vi "Translate Data to Virtual Device Data.vi"(10 "HVAC Data":T1) -> (1 "Data Array":u16[](array[numeric]), 2 "Address":u16)   [LabVIEW 2015, in "SLZ-KA1 Actor.lvlib" / "SLZ-KA1.lvclass"]
doc: "This code converts the data coming from the real device to the format the EMS understands."
uses:
  SLZ-KA1.lvclass
  Controls/SLZ-KA1 Real Data Cluster.ctl
  Utilities/Modbus Data Conversion.llb/Modbus Data Conversion.lvlib
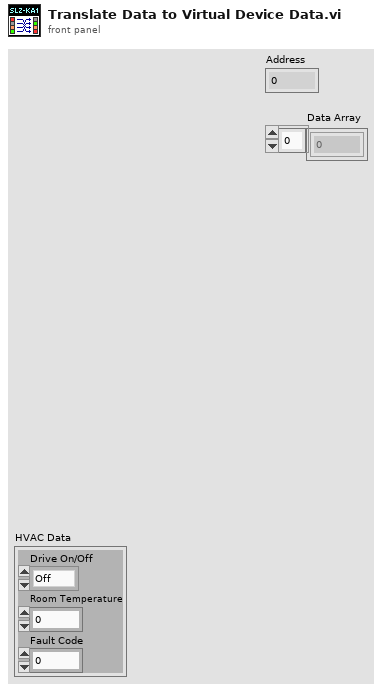
[diagram p1: front panel]
types:
  T1 = typedef "SLZ-KA1 Actor.lvlib/SLZ-KA1.lvclass/SLZ-KA1 Real Data Cluster.ctl" = cluster{"Drive On/Off":enum16{"Off", "On"}, "Room Temperature":dbl, "Fault Code":u16}
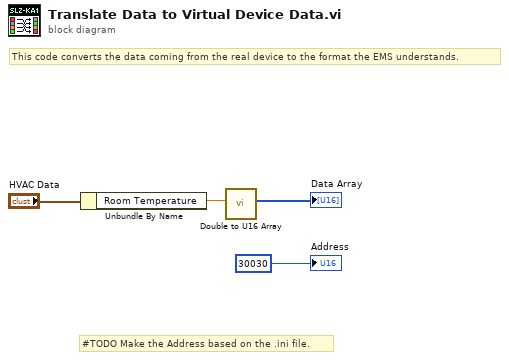
[diagram p0: block diagram]
diagram:
  # "This code converts the data coming from the real device to the format the EMS understands."
  # "#TODO Make the Address based on the .ini file."
  n1 = Unbundle By Name("HVAC Data") -> ("Room Temperature"=w1:dbl)
  n2 = call "Double to U16 Array.vi"("Double"=w1) -> ("U16 Array"=→"Data Array":u16[])  [unwired: 10 in]
  "Address" <- u16 30030 ("Address")
